vi "XL320_Scan for Motors by Ping.vi"(0 "VISA resource name":refnum<visa-resource-name>, 5 "Starting ID (0)":u8, 7 "Ending ID (252)":u8=252, 9 "Search Timeout (10000 ms)":u32=10000, 11 "error in (no error)":errorcluster) -> (4 "VISA resource name out":refnum<visa-resource-name>, 6 "Motors IDs Found":u8[](array[numeric]), 15 "error out":errorcluster)   [LabVIEW 2015, in "Dynamixel XL320.lvlib"]
doc: "Scans sequentially for motors between <b>Starting ID</b> and <b>Ending ID</b> for no longer than <b>Search Timeout</b>. If all of the motors do not have unique IDs, then motors with duplicate IDs may not be found."
uses:
  <instrlib>/Dynamixel XL320/Dynamixel XL320.lvlib
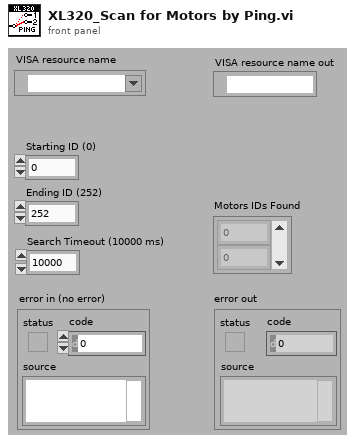
[diagram p1: front panel]
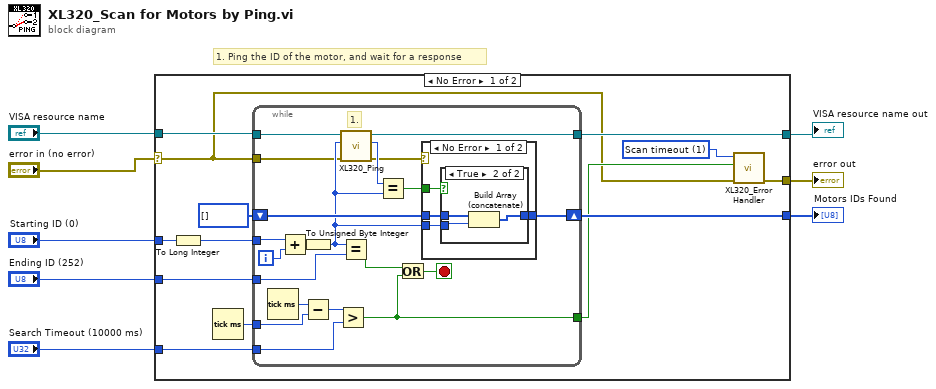
[diagram p0: block diagram]
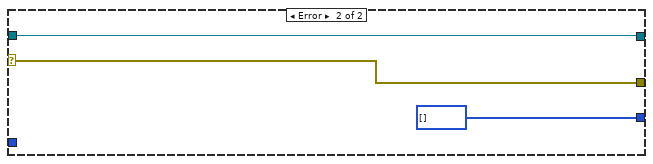
[diagram p4: hidden frame]
diagram:
  # "1. Ping the ID of the motor, and wait for a response"
  n1 = case shown="No Error" "error in (no error)" {
    selector: "error in (no error)" -> [w10 w53]
    tunnel: "VISA resource name" -> [w15 w52]
    tunnel: [w21 w52] -> w4
    tunnel: [w9 w53] -> w5
    tunnel: [w17 u8[] []] -> w8
    tunnel: "Starting ID (0)" -> [w20 _]
    tunnel: "Ending ID (252)" -> [w18 _]
    tunnel: "Search Timeout (10000 ms)" -> [w13 _]
    frame No Error {
      w12 = u16 1 items=["Default (no error)", "Scan timeout", "Invalid motor checksum", "Unexpected return string", "Invalid address range"] ("Error type")
      n2 = To Long Integer(number=w20) -> (32bit integer=w16:i32)
      n3 = Tick Count (ms)() -> (millisecond timer value=w14:u32)
      n4 = while {
        tunnel: w15 -> [w26]
        shift-right: [w37] -> w17
        shift-left: u8[] [] -> [w39]
        tunnel: [w27] -> w21
        tunnel: w10 -> [w24]
        tunnel: w16 -> [w35]
        tunnel: w18 -> [w34]
        tunnel: w14 -> [w31]
        tunnel: w13 -> [w29]
        tunnel: [w28] -> w11
        i -> [w41]
        stop <- w36 stop-if-true
        # "1."
        n5 = Tick Count (ms)() -> (millisecond timer value=w32:u32)
        n6 = Add(x=w35, y=w41) -> (x+y=w38:i32)
        n7 = To Unsigned Byte Integer(number=w38) -> (unsigned 8bit integer=w25:u8)
        n8 = Subtract(x=w32, y=w31) -> (x-y=w30:u32)
        n9 = Greater?(x=w30, y=w29) -> (0:w28:bool)
        n10 = call <instrlib>:"XL320_Ping.vi"("error in (no error)"=w24, "Motor ID"=w25, "VISA Refnum in"=w26) -> ("error out"=w22:errorcluster, "Motor ID out"=w23:u8, "VISA Refnum out"=w27:refnum<visa-resource-name>)  [unwired: 6 in]
        n11 = Equal?(x=w25, y=w34) -> (x = y?=w33:bool)
        n12 = Equal?(x=w23, y=w25) -> (x = y?=w40:bool)
        n13 = Or(x=w33, y=w28) -> (x .or. y?=w36:bool)
        n14 = case shown="No Error" w22 {
          tunnel: w40 -> [w45 _]
          tunnel: w39 -> [w44 w50]
          tunnel: [w43 w50] -> w37
          tunnel: w25 -> [w42 _]
          frame No Error {
            n15 = case shown="True" w45 {
              tunnel: w44 -> [w46 w49]
              tunnel: w42 -> [_ w48]
              tunnel: [w46 w47] -> w43
              frame False {
              }
              frame True {
                n16 = Build Array (concatenate)(w49, w48) -> (w47:u8[])
              }
            }
          }
          frame Error {
          }
        }
      }
      n17 = call <instrlib>:"XL320_Error Handler.vi"("error in (no error)"=w10, "Error? (no error)"=w11, "Error type"=w12) -> ("error out"=w9:errorcluster)  [unwired: 8 in]
    }
    frame Error {
    }
  }
  "Motors IDs Found" <- w8
  "error out" <- w5
  "VISA resource name out" <- w4
